vi "GPM Repo URL--constant.vi"() -> (3 "GPM Repo URL":string)   [LabVIEW 2016, in "Packages.lvlib" / "GPM.lvlib"]
uses:
  GPM.lvlib
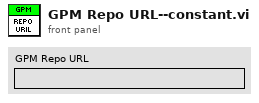
[diagram p1: front panel]
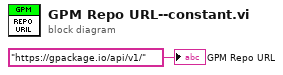
[diagram p0: block diagram]
diagram:
  "GPM Repo URL" <- "https://gpackage.io/api/v1/"
